vi "Test-Host-CryptoNight-Step-3.vi"() -> ()   [LabVIEW 2017]
panel:
  out "Values Match? 2":bool
  out "Values Match?":bool
  out "exp_hp_state_out":u8[](array[numeric]) format="%.0x"
  out "Runtime (minutes)":dbl
  in  "Override Iterations":bool
  out "Runtime (s)":dbl
  out "Runtime (ms)":u32
  in  "# of Iterations":i32
  out "hp_state out":u8[](array[numeric]) format="%.0x"
  out "b_out":u64[](array[numeric]) format="%.0x"
  out "a_out":u64[](array[numeric]) format="%.0x"
  in  "FileName":string="log_file.8.bin"
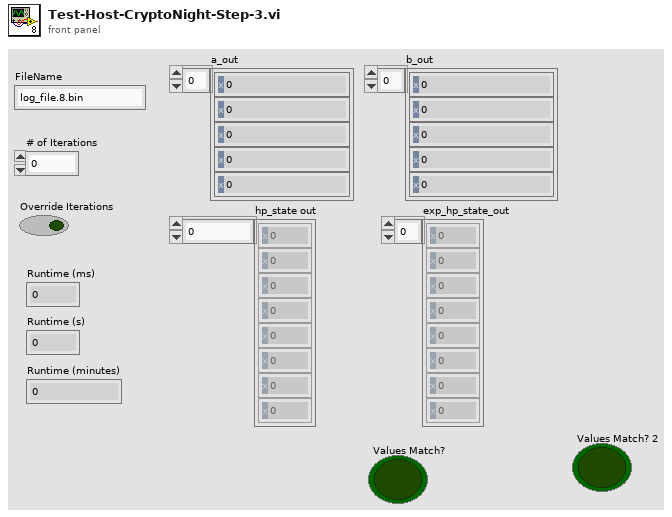
[diagram p1: front panel]
types:
  T1 = typedef "Step-3-Data-Type.ctl" = cluster{"a":u64[], "b":u64[], "hp_state_in":u8[], "hp_state_out":u8[], "hp_state_in (u64)":u64[], "hp_state_out (u64)":u64[]}
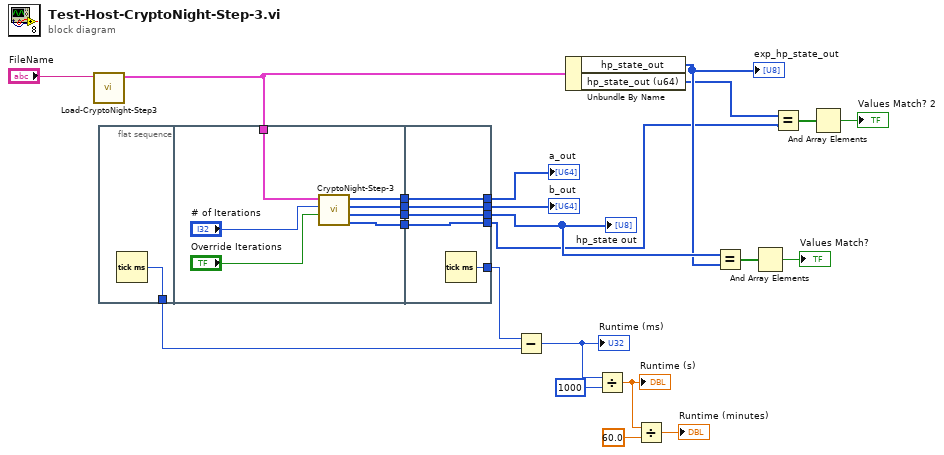
[diagram p0: block diagram]
diagram:
  n1 = call "Load-CryptoNight-Step3.vi"("FileName"="FileName") -> ("output cluster"=w8:T1)  [unwired: 9 in, 1 out]
  n2 = flat-sequence {
    tunnel: [w24] -> w17
    tunnel: [w31] -> w21
    tunnel: [w30] -> w20
    tunnel: [w29] -> w19
    tunnel: w8 -> [w26]
    tunnel: [w25] -> w5
    tunnel: [w34] -> w11
    tunnel: [w35] -> w22
    tunnel: [w36] -> w23
    tunnel: w21 -> [w36]
    tunnel: w20 -> [w35]
    tunnel: w19 -> [w34]
    tunnel: [w33] -> w18
    tunnel: [w32] -> w2
    tunnel: w5 -> [w32]
    frame #0 {
      n3 = Tick Count (ms)() -> (millisecond timer value=w24:u32)
    }
    frame #1 {
      n4 = call "CryptoNight-Step-3.vi"("Override Iterations"="Override Iterations", "# of Iterations"="# of Iterations", "input"=w26) -> ("hp_state out (u64)"=w25:u64[], "hp_state out"=w29:u8[], "b_out"=w30:u64[], "a_out"=w31:u64[])  [unwired: 5 in]
    }
    frame #2 {
      n5 = Tick Count (ms)() -> (millisecond timer value=w33:u32)
    }
  }
  n6 = Subtract(x=w18, y=w17) -> (x-y=w16:u32)
  "Runtime (ms)" <- w16
  n7 = Unbundle By Name(w8) -> ("hp_state_out"=w6:u8[], "hp_state_out (u64)"=w1:u64[])
  "exp_hp_state_out" <- w6
  n8 = Divide(x=w16, y=u32 1000) -> (x/y=w14:dbl)
  "Runtime (s)" <- w14
  n9 = Divide(x=w14, y=60.0) -> (x/y=→"Runtime (minutes)":dbl)
  n10 = Equal?(x=w11, y=w6) -> (x = y?=w10:bool[])
  n11 = And Array Elements(Boolean array=w10) -> (logical AND=→"Values Match?":bool)
  n12 = Equal?(x=w1, y=w2) -> (x = y?=w4:bool[])
  n13 = And Array Elements(Boolean array=w4) -> (logical AND=→"Values Match? 2":bool)
  "a_out" <- w23
  "b_out" <- w22
  "hp_state out" <- w11
